vi "91 WIO_Reading a voltage.vi"() -> ()   [LabVIEW 2019]
uses:
  <vilib>/httpClient/LabVIEWHTTPClient.lvlib
  _Subs/OpenDiagram/Open_XControl.xctl
panel:
  in  "OpenDiag":refnum<vi>(xcontrol)
  out "Temperature":dbl(knob) scale=0.0..100.0
  # "01 Reading a Voltage\nThis code reads the temperature from your WIO Link\n\nInstructions:\n1. Connect up your WIO to the cloud with the phone app\n       (see http://iot.seeed.cc)\n2. Configure it to measure temperature\n3. Use LabVIEW to read the last temperature reading (enter access_token in diagram)\n       (you can get your token from the app under view API)\n4. Hit continuous run to see the temperature change"
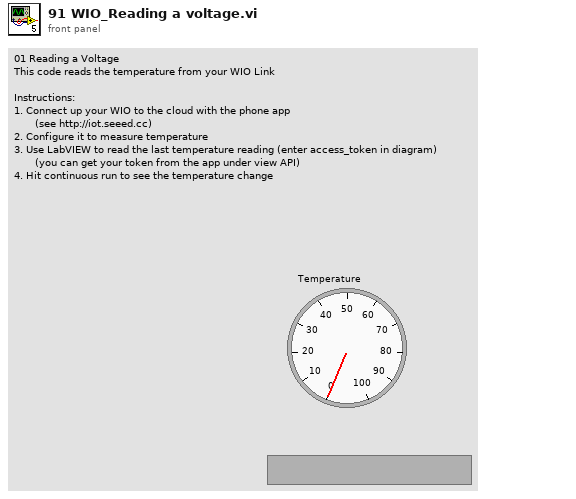
[diagram p1: front panel]
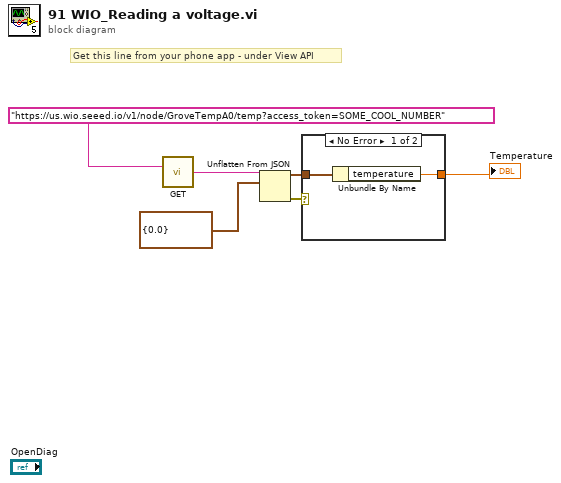
[diagram p0: block diagram]
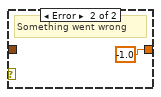
[diagram p2: hidden frame]
diagram:
  # "Get this line from your phone app - under View API"
  n1 = call <vilib>:"GET.vi"("url"="https://us.wio.seeed.io/v1/node/GroveTempA0/temp?access_token=SOME_COOL_NUMBER") -> ("body"=w3:string)  [unwired: 11 in, 3 out]
  n2 = Unflatten From JSON(JSON string=w3, type and defaults=cluster{"temperature":dbl} {"temperature"=0.0}) -> (value=w5:cluster{"temperature":dbl}, error out=w4:errorcluster)  [unwired: 5 in]
  n3 = case shown="No Error" w4 {
    tunnel: w5 -> [w8 _]
    tunnel: [w7 -1.0 ("temperature")] -> w1
    frame No Error {
      n4 = Unbundle By Name(w8) -> ("temperature"=w7:dbl)
    }
    frame Error {
      # "Something went wrong"
    }
  }
  "Temperature" <- w1
